vi "pitch_roll.vi"(8 "flipperbob":bool, 9 "Az":dbl, 10 "Ay":dbl, 11 "Ax":dbl) -> (1 "Pitch":dbl, 3 "Roll":dbl)   [LabVIEW 2009]
panel:
  out "regular pitch":dbl
  out "rolled over?":bool
  out "regular roll":dbl
  out "not pitched up?":bool
  out "regular roll":dbl
  out "x .and. y?":bool
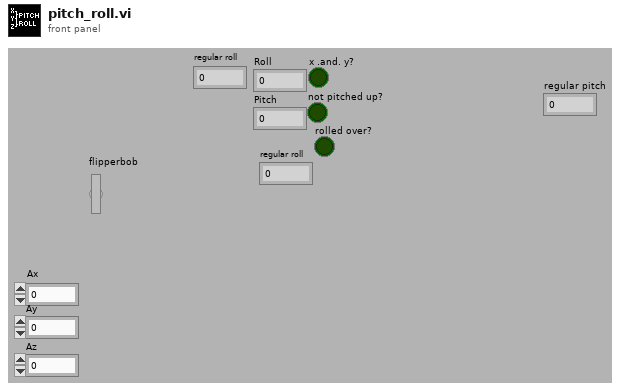
[diagram p1: front panel]
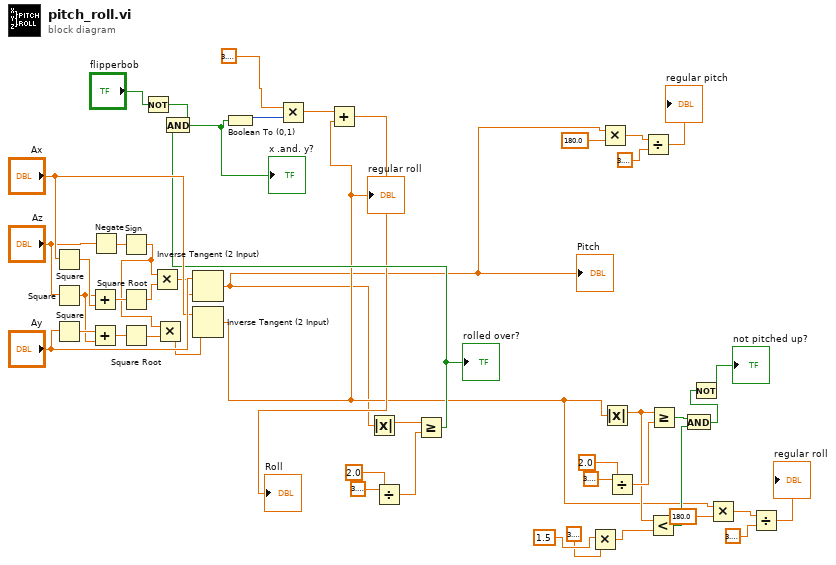
[diagram p0: block diagram]
diagram:
  n1 = Square(x="Ax") -> (x^2=w47:dbl)
  n2 = Square(x="Az") -> (x^2=w42:dbl)
  n3 = Square(x="Ay") -> (x^2=w43:dbl)
  n4 = Add(x=w42, y=w47) -> (x+y=w46:dbl)
  n5 = Add(x=w43, y=w42) -> (x+y=w44:dbl)
  n6 = Negate(x="Az") -> (-x=w35:dbl)
  n7 = Sign(1:w35) -> (0:w1:dbl)
  n8 = Square Root(x=w46) -> (sqrt(x)=w40:dbl)
  n9 = Square Root(x=w44) -> (sqrt(x)=w39:dbl)
  n10 = Not(x="flipperbob") -> (.not. x?=w29:bool)
  n11 = Multiply(x=w1, y=w40) -> (x*y=w37:dbl)
  n12 = Multiply(x=w1, y=w39) -> (x*y=w38:dbl)
  n13 = Inverse Tangent (2 Input)(1:w37, 2:"Ay") -> (0:w3:dbl)
  "Pitch" <- w3
  n14 = Inverse Tangent (2 Input)(1:w38, 2:"Ax") -> (0:w8:dbl)
  "regular roll" <- w8
  n15 = Absolute Value(x=w3) -> (abs(x)=w24:dbl)
  n16 = Divide(x=3.141592653589793, y=2.0) -> (x/y=w31:dbl)
  n17 = Greater Or Equal?(x=w24, y=w31) -> (x >= y?=w28:bool)
  "rolled over?" <- w28
  n18 = And(x=w29, y=w28) -> (x .and. y?=w2:bool)
  "x .and. y?" <- w2
  n19 = Boolean To (0,1)(Boolean=w2) -> (0, 1=w34:i16)
  n20 = Multiply(x=3.141592653589793, y=w34) -> (x*y=w27:dbl)
  n21 = Add(x=w27, y=w8) -> (x+y=→"Roll":dbl)
  n22 = Multiply(x=1.5 ("y"), y=3.141592653589793) -> (x*y=w19:dbl)
  n23 = Multiply(x=w3, y=180.0) -> (x*y=w6:dbl)
  n24 = Absolute Value(x=w8) -> (abs(x)=w12:dbl)
  n25 = Divide(x=3.141592653589793, y=2.0) -> (x/y=w21:dbl)
  n26 = Divide(x=w6, y=3.141592653589793) -> (x/y=→"regular pitch":dbl)
  n27 = Less?(x=w12, y=w19) -> (x < y?=w14:bool)
  n28 = Greater Or Equal?(x=w12, y=w21) -> (x >= y?=w16:bool)
  n29 = And(x=w16, y=w14) -> (x .and. y?=w15:bool)
  n30 = Not(x=w15) -> (.not. x?=→"not pitched up?":bool)
  n31 = Multiply(x=w8, y=180.0) -> (x*y=w11:dbl)
  n32 = Divide(x=w11, y=3.141592653589793) -> (x/y=→"regular roll":dbl)
